vi "Init.vi"(8 "error in (no error)":errorcluster, 10 "Instrument String":variant, 11 "NI-Sync in":refnum<class "NI-Sync.lvclass">) -> (0 "error out":errorcluster, 2 "Found?":bool, 3 "NI-Sync out":refnum<class "NI-Sync.lvclass">)   [LabVIEW 2025, in "Synchronization.lvlib" / "NI-Sync.lvclass"]
uses:
  NI-Sync.lvclass
  C:/Working copy/tss/Plugin/Engines/Synchronization/Synchronization Instrument/Synchronization Instrument.lvclass
  Synchronization configuration/Synchronization configuration.lvclass
  C:/Users/Public/Documents/Sandia National Labs/TSS Plugin/Abstract Engine.lvlibp/Plugin/Abstract/Instrument configuration/Instrument configuration.lvclass
  NI-Sync.lvclass/NI-Sync.ctl
  Users/Public/Documents/Sandia National Labs/TSS Plugin/Abstract Engine.lvlibp/Plugin/Abstract/Instrument configuration/Read Instrument Setting.vi
  <instrlib>/niSync/niSync.llb/niSync Initialize (Default).vi
  Users/Public/Documents/Sandia National Labs/TSS Plugin/CEF.lvlibp/serializable configuration/CEF_serializable configuration.lvclass
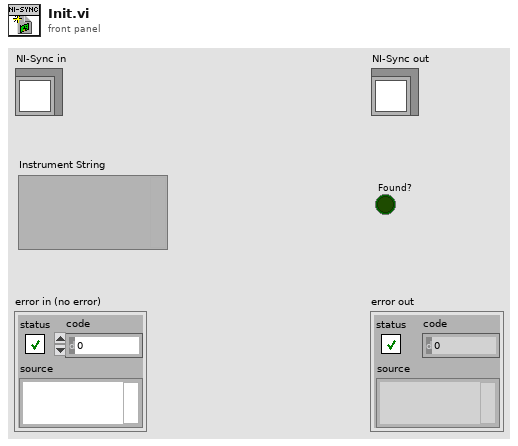
[diagram p1: front panel]
types:
  T1 = typedef "Abstract Engine.lvlibp/Instrument configuration.lvclass/Default Instrument.ctl" = cluster{"Type":string, "Address":string, "SW Alias":string, "Description":string, "Enabled":bool}
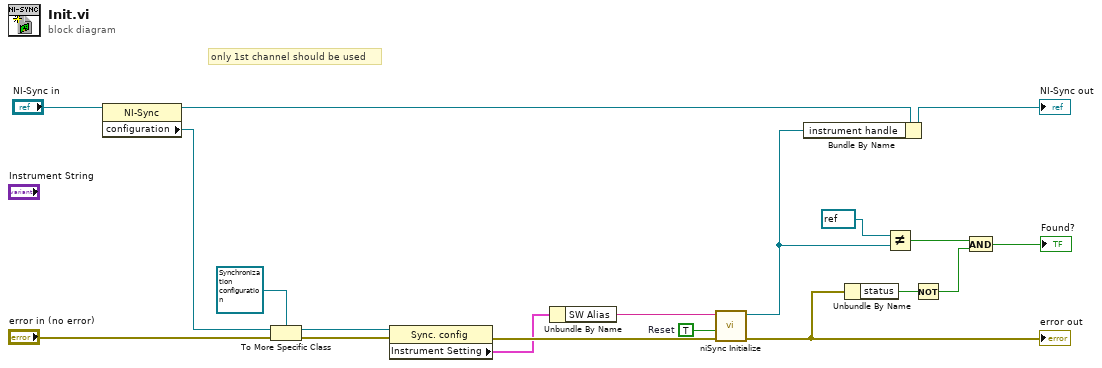
[diagram p0: block diagram]
diagram:
  w11 = TRUE  # Reset
  # "only 1st channel should be used"
  n1 = property class="NI-Sync"(reference="NI-Sync in") -> (reference out=w17:refnum<class "NI-Sync.lvclass">, "configuration"=w15:refnum<class "CEF_serializable configuration.lvclass">)  [unwired: 1 in, 1 out]
  n2 = To More Specific Class(target class=refnum<class "Synchronization configuration.lvclass"> refnum ("DMM.lvlib:DMM configuration.lvclass"), reference=w15, error in="error in (no error)") -> (specific class reference=w16:refnum<class "Synchronization configuration.lvclass">, error out=w13:errorcluster)
  n3 = property class="Sync. config"(reference=w16, error in=w13) -> (error out=w10:errorcluster, "Instrument Setting"=w6:T1)  [unwired: 1 out]
  n4 = Unbundle By Name(w6) -> ("SW Alias"=w9:string)
  n5 = call-poly <instrlib>:"niSync Initialize.vi"("error in (no error)"=w10, "reset device (F)"=w11, "resource name"=w9) -> ("error out"=w4:errorcluster, "instrument handle out"=w8:refnum<k15>)  [unwired: 7 in]
  "error out" <- w4
  n6 = Bundle By Name(cluster=w17, "instrument handle"=w8) -> (→"NI-Sync out":refnum<class "NI-Sync.lvclass">)
  n7 = Unbundle By Name(w4) -> ("status"=w3:bool)
  n8 = Not Equal?(x=refnum<k15> refnum ("instrument handle out"), y=w8) -> (x != y?=w2:bool)
  n9 = Not(x=w3) -> (.not. x?=w5:bool)
  n10 = And(x=w2, y=w5) -> (x .and. y?=→"Found?":bool)
